vi "AccelerometerVoltageSampleLoop.vi"   [LabVIEW 2016]
uses:
  AccelerometerSample.ctl
  <vilib>/rvi/Emulation/niFpgaGetClockAttributes.vi
  <vilib>/rvi/Emulation/niFpgaSctlEmulationGetInTimedLoop.vi
  <vilib>/rvi/Emulation/niFpgaEmulationReportErrorSimple.vi
  <vilib>/rvi/Emulation/niFpgaEmulationIsFPGAContextNoSignature.vi
  <vilib>/rvi/errors/niFpgaSetErrorForExecOnDevCompSimple.vi
  <vilib>/rvi/eio/common/nirviEmuReportErrorAndStop.vi
  <vilib>/rvi/DataTransferAndStorage/Container/Common/niFpgaContainerGetUniqueNameForEmu.vi
  <vilib>/rvi/FIFO/Fifo_Resource/nirvififoEmulationSetSize.vi
  <vilib>/rvi/FIFO/Fifo_Resource/nirviFifoEmulationQueueMgr.vi
  <instcachedir>/0/nirviFifoEmulationQueueMgr_E5CAEC123FF24DC58D834DCA3CDAA9B5.lvgen/nirviFifoEmulationQueueMgr_E5CAEC123FF24DC58D834DCA3CDAA9B5_004.vi
  <vilib>/Utility/error.llb/Clear Errors.vi
  <vilib>/rvi/FIFO/Fifo_Resource/nirvififoEmulationCreateLock.vi
  <vilib>/rvi/Emulation/niFpgaProcessEmulError.vi
  <vilib>/rvi/FIFO/Fifo_Resource/nirvififoEmulationObtainLock.vi
  <vilib>/rvi/FIFO/Fifo_Resource/nirvififoEmulationReleaseLock.vi
  <vilib>/rvi/occurrence/nirviWaitOnOccurrenceBase.vi
  <vilib>/rvi/errors/nirviReportUnexpectedCaseInternalError.vi
  <vilib>/rvi/errors/nirviReportUnexpectedCaseInternalError (U32).vi
  <vilib>/rvi/eio/common/nirviEmuTemplateMethod_errors.vi
  <instcachedir>/0/nirviFifoEmulationQueueMgr_E5CAEC123FF24DC58D834DCA3CDAA9B5.lvgen/nirviFifoEmulationQueueMgr_E5CAEC123FF24DC58D834DCA3CDAA9B5_026.vi
  <vilib>/rvi/FIFO/Fifo_Resource/nirvififoEmulationDetermineInputValidOut.vi
  <vilib>/rvi/Emulation/niFpgaCriticalErrorInLSC.vi
  <vilib>/rvi/DataTransferAndStorage/Container/XNode/niFpgaContainer.xnode
  <vilib>/rvi/FIFO/Fifo_Resource/nirvififoEmulationRead.vi
  <vilib>/eio/EIONode/EIONode.xnode
  <vilib>/rvi/FIFO/Fifo_Resource/nirvififoEmulationWrite.vi
types:
  T1 = typedef "AccelerometerSample.ctl" = cluster{"Timestamp":u64, "Accelerometer1Voltage":sgl, "Accelerometer2Voltage":sgl, "Accelerometer3Voltage":sgl, "Accelerometer4Voltage":sgl, "Accelerometer5Voltage":sgl, "Accelerometer6Voltage":sgl, "Accelerometer7Voltage":sgl, "Accelerometer8Voltage":sgl, "Accelerometer1Acceleration":sgl, "Accelerometer2Acceleration":sgl, "Accelerometer3Acceleration":sgl, "Accelerometer4Acceleration":sgl, "Accelerometer5Acceleration":sgl, "Accelerometer6Acceleration":sgl, "Accelerometer7Acceleration":sgl, "Accelerometer8Acceleration":sgl, "AngularAccelerationX":sgl, "AngularAccelerationY":sgl, "AngularAccelerationZ":sgl}
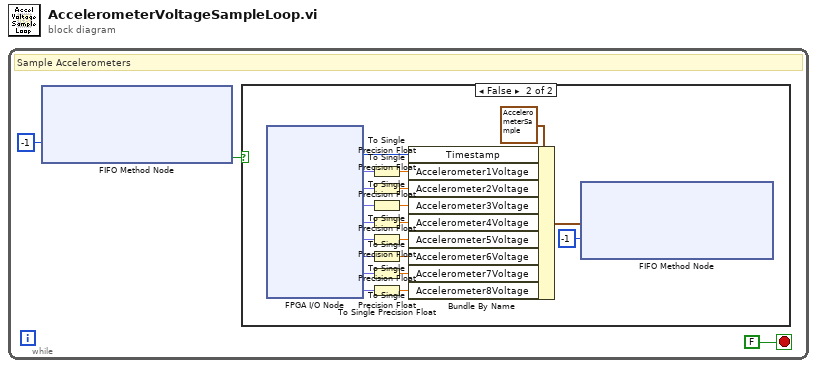
[diagram p0: block diagram]
diagram:
  n1 = while {
    stop <- FALSE stop-if-true
    # "Sample Accelerometers"
    n2 = xnode ("FIFO Method Node")("Timeout"=-1) -> ("Timed Out?"=w2:bool)  [unwired: 1 in, 2 out]
    n3 = case shown="False" w2 {
      frame True {
      }
      frame False {
        n4 = xnode "FPGA I/O Node"() -> ("Time"=w15:u64, "Mod1/AI0"=w23:fxp<+/-,24,5>, "Mod1/AI1"=w22:fxp<+/-,24,5>, "Mod1/AI2"=w21:fxp<+/-,24,5>, "Mod1/AI3"=w20:fxp<+/-,24,5>, "Mod2/AI0"=w19:fxp<+/-,24,5>, "Mod2/AI1"=w18:fxp<+/-,24,5>, "Mod2/AI2"=w17:fxp<+/-,24,5>, "Mod2/AI3"=w16:fxp<+/-,24,5>)  [unwired: 9 in, 9 out]
        n5 = To Single Precision Float(number=w23) -> (single precision float=w14:sgl)
        n6 = To Single Precision Float(number=w22) -> (single precision float=w13:sgl)
        n7 = To Single Precision Float(number=w21) -> (single precision float=w12:sgl)
        n8 = To Single Precision Float(number=w20) -> (single precision float=w11:sgl)
        n9 = To Single Precision Float(number=w19) -> (single precision float=w10:sgl)
        n10 = To Single Precision Float(number=w18) -> (single precision float=w9:sgl)
        n11 = To Single Precision Float(number=w17) -> (single precision float=w8:sgl)
        n12 = To Single Precision Float(number=w16) -> (single precision float=w7:sgl)
        n13 = Bundle By Name(cluster=T1 {"Timestamp"=0, "Accelerometer1Voltage"=0.0, "Accelerometer2Voltage"=0.0, "Accelerometer3Voltage"=0.0, "Accelerometer4Voltage"=0.0, "Accelerometer5Voltage"=0.0, "Accelerometer6Voltage"=0.0, "Accelerometer7Voltage"=0.0, "Accelerometer8Voltage"=0.0, "Accelerometer1Acceleration"=0.0, "Accelerometer2Acceleration"=0.0, "Accelerometer3Acceleration"=0.0, "Accelerometer4Acceleration"=0.0, "Accelerometer5Acceleration"=0.0, "Accelerometer6Acceleration"=0.0, "Accelerometer7Acceleration"=0.0, "Accelerometer8Acceleration"=0.0, "AngularAccelerationX"=0.0, "AngularAccelerationY"=0.0, "AngularAccelerationZ"=0.0} ("AccelerometerSample"), "Timestamp"=w15, "Accelerometer1Voltage"=w14, "Accelerometer2Voltage"=w13, "Accelerometer3Voltage"=w12, "Accelerometer4Voltage"=w11, "Accelerometer5Voltage"=w10, "Accelerometer6Voltage"=w9, "Accelerometer7Voltage"=w8, "Accelerometer8Voltage"=w7) -> (w6:T1)
        n14 = xnode ("FIFO Method Node")("Element"=w6, "Timeout"=-1) -> ()  [unwired: 1 in, 2 out]
      }
    }
  }
